vi "Wait-for-action-Process1.vi"(8 "error in (no error)":errorcluster, 11 "Object ref in":T2) -> (0 "error out":errorcluster, 2 "Action":T1, 3 "Object ref out":T2)   [LabVIEW 2013, in "HardwareCharacterization.lvlib" / "HC-Main.lvclass"]
uses:
  HC-Main.lvclass
  Object-reference.ctl
  Process1-actions.ctl
  HC-Main.lvclass/HC-Main.ctl
  Read Process 1 queue.vi
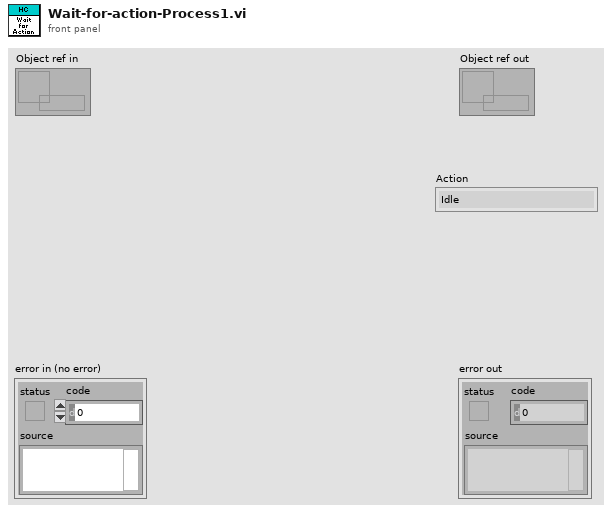
[diagram p1: front panel]
types:
  T1 = typedef "HardwareCharacterization.lvlib/HC-Main.lvclass/Process1-actions.ctl" = enum16{"Idle", "Activate", "Analyse scan file", "Convert SM1000positions", "Measure SM1000 timings", "Measure laser timings", "Stop", "Abort", "Exit"}
  T2 = typedef "HardwareCharacterization.lvlib/HC-Main.lvclass/Object-reference.ctl" = refnum<data-value>
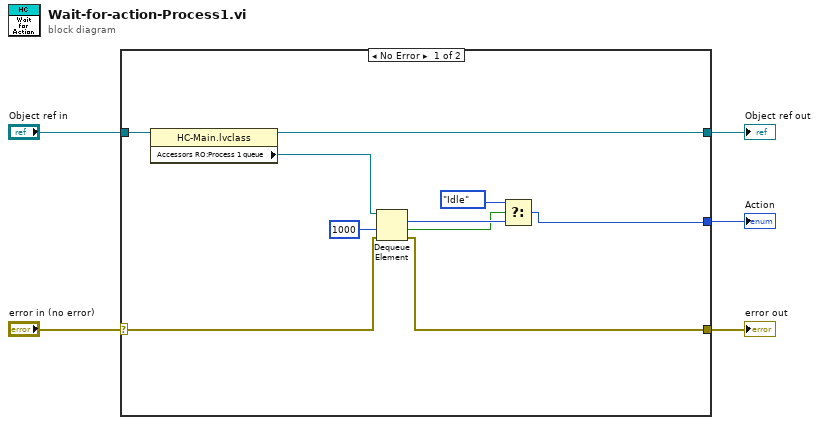
[diagram p0: block diagram]
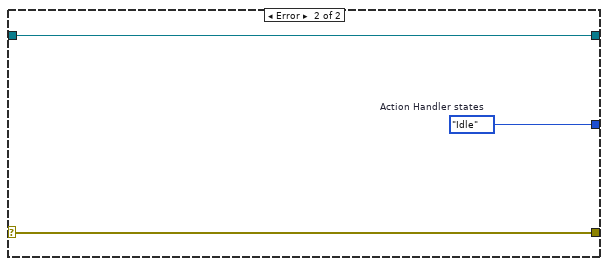
[diagram p2: hidden frame]
diagram:
  n1 = case shown="No Error" "error in (no error)" {
    selector: "error in (no error)" -> [w13 w18]
    tunnel: [w12 w18] -> w4
    tunnel: [w14 w17] -> w2
    tunnel: "Object ref in" -> [w15 w17]
    tunnel: [w6 w16] -> w1
    frame No Error {
      n2 = property class="HC-Main.lvclass"(reference=w15) -> (reference out=w14:T2, "Accessors RO:Process 1 queue"=w11:refnum<queue>)  [unwired: 1 in, 1 out]
      n3 = Dequeue Element(queue=w11, timeout in ms (-1)=1000, error in (no error)=w13) -> (element=w9:T1, timed out?=w8:bool, error out=w12:errorcluster)  [unwired: 1 out]
      n4 = Select(t=Process1-actions."Idle" ("Next execution"), s=w8, f=w9) -> (s? t:f=w6:T1)
    }
    frame Error {
      w16 = Process1-actions."Idle"  # Action Handler states
    }
  }
  "error out" <- w4
  "Object ref out" <- w2
  "Action" <- w1
